vi "MFC-2000 Stage Engine.vi"(0 "MS-2000 Notifier Name":string="MS2000", 11 "COM Port":string[](array[string])) -> ()   [LabVIEW 2020]
uses:
  Stages Controls/Stage Notifier Element.ctl
  Stages Controls/Stage Actions.ctl
  Stages Controls/Stage Status.ctl
  <vilib>/Instr/_visa.llb/VISA Configure Serial Port (Instr).vi
panel:
  in  "XY Velocity (µm/s)":dbl format="%#_4g"
  out "Reply":string
  in  "Command":string
  out "Last Error":errorcluster
  in  "Get Position":bool
  in  "XY Step Size (µm)":dbl format="%#_4g"
  in  "Y Position (µm)":dbl format="%#_4g"
  in  "X Position (µm)":dbl format="%#_4g"
  in  "Home":bool
  in  "Right":bool
  in  "Left":bool
  in  "Down":bool
  in  "Halt":bool
  in  "Up":bool
  in  "Quit":bool
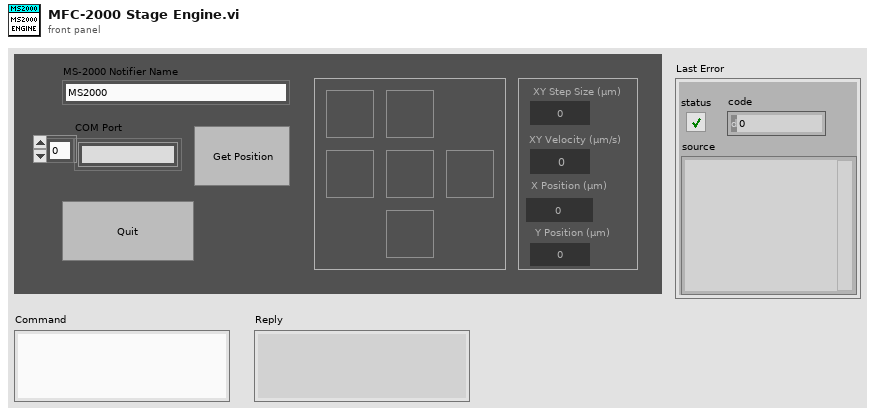
[diagram p1: front panel]
types:
  T1 = typedef "Stage Notifier Element.ctl" = cluster{"Action":T2, "Axis":bool[], "Setpoint":dbl[], "Velocity":dbl, "Cmd Recvd?":bool, "Position":dbl[], "Status":T3, "Misc":variant}
  T2 = typedef "Stage Actions.ctl" = enum16{"Get Position", "MVR", "MOVE", "HALT", "ONTARGET", "ERROR", "REFERENCE", "INIT", "VELOCITY", "STATUS", "EXIT", "HOME", "ZEROPOS", "NANOPOS", "ANALOG", "QUIT"}
  T3 = typedef "Stage Status.ctl" = enum16{"Error", "Abort", "Busy", "On Target"}
  T4 = enum32{"Invalid", "Standard", "Closed", "Hidden", "Minimized", "Maximized"}
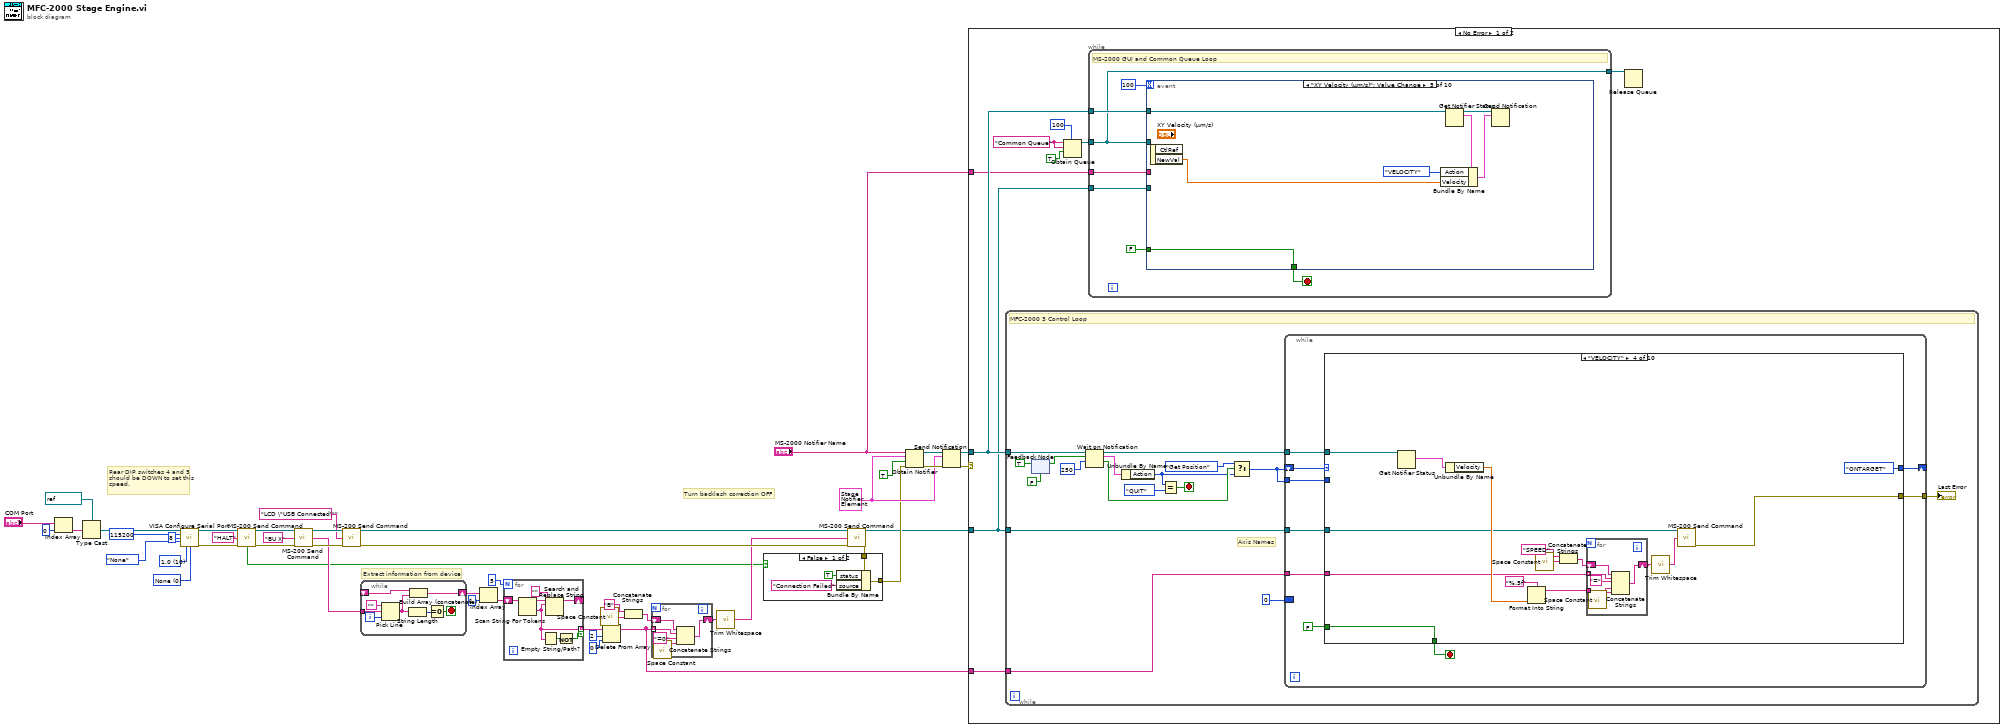
[diagram p0: block diagram]
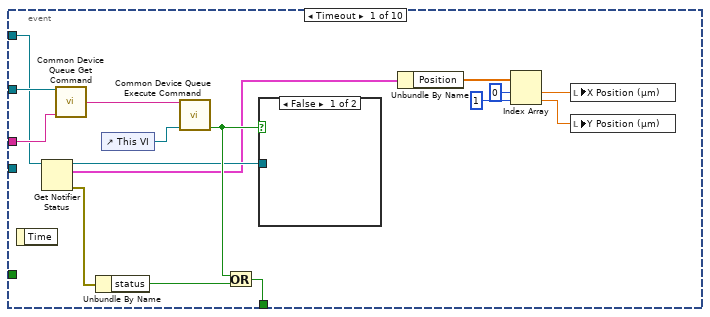
[diagram p3: hidden frame]
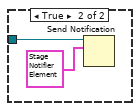
[diagram p4: hidden frame]
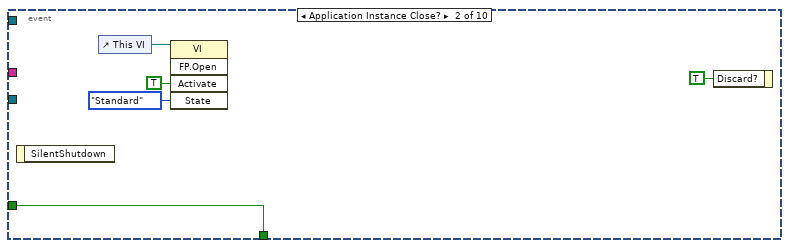
[diagram p5: hidden frame]
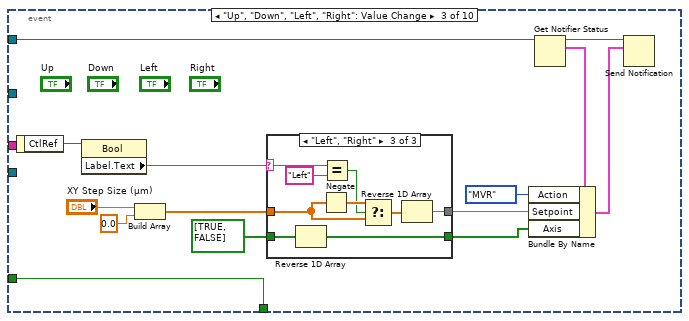
[diagram p6: hidden frame]
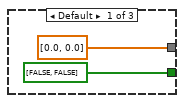
[diagram p7: hidden frame]
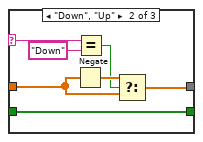
[diagram p8: hidden frame]
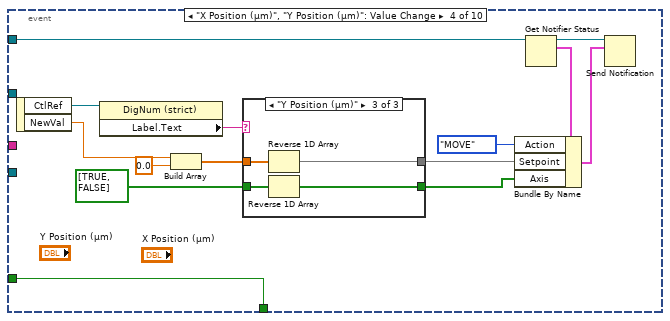
[diagram p9: hidden frame]
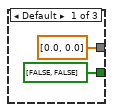
[diagram p10: hidden frame]
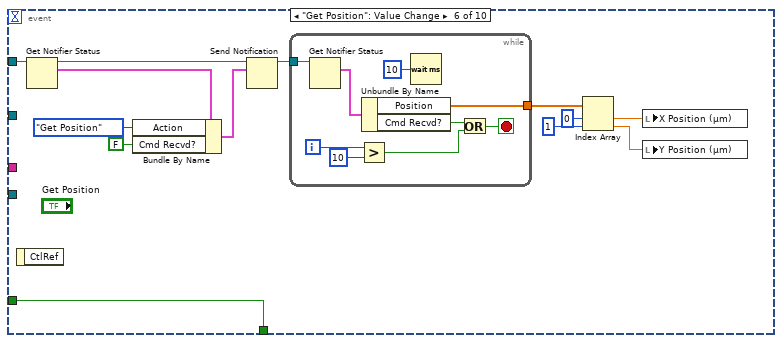
[diagram p12: hidden frame]
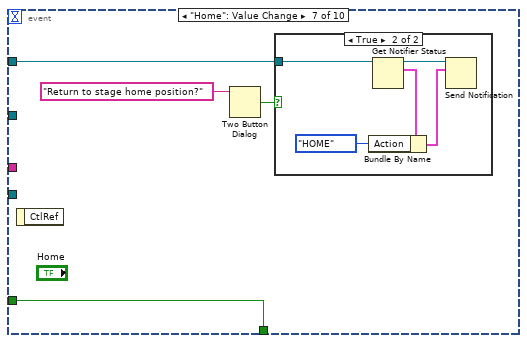
[diagram p13: hidden frame]
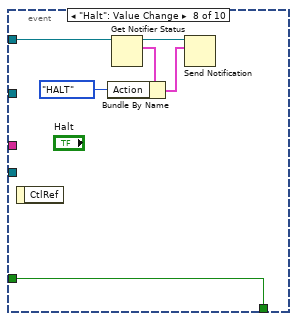
[diagram p15: hidden frame]
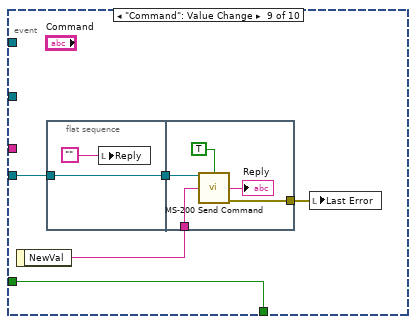
[diagram p16: hidden frame]
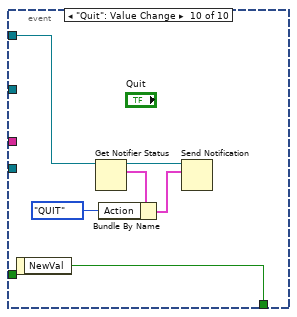
[diagram p17: hidden frame]
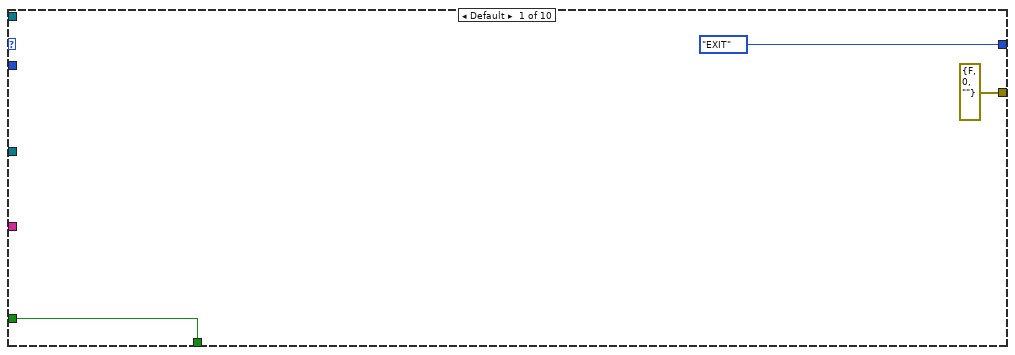
[diagram p18: hidden frame]
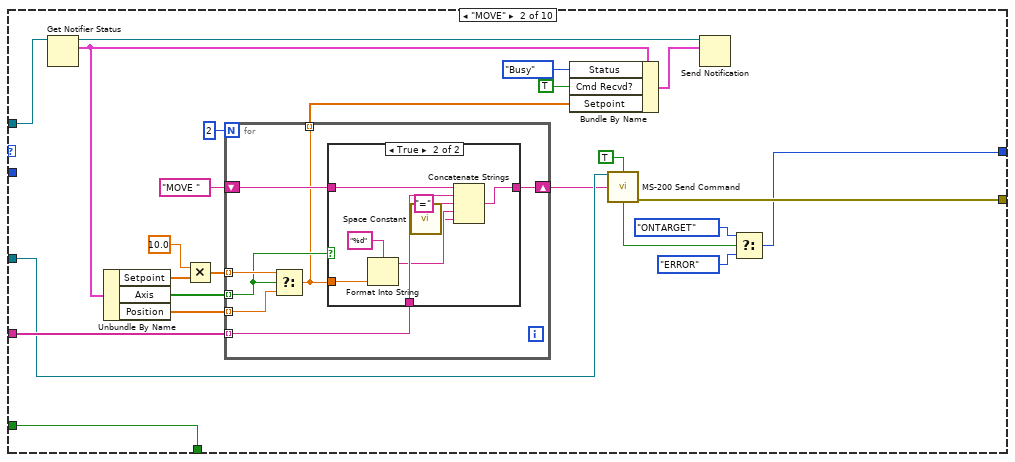
[diagram p19: hidden frame]
diagram:
  w37 = u16 0 items=["None", "XON/XOFF", "RTS/CTS", "XON/XOFF & RTS/CTS", "DTR/DSR", "XON/XOFF & DTR/DSR"] ("flow control (0:none)")
  w39 = u16 10 items=["1.0"=10, "1.5"=15, "2.0"=20] ("stop bits (10: 1 bit)")
  w41 = T1 {"Action"=enum."Get Position", "Axis"=[], "Setpoint"=[], "Velocity"=0.5, "Cmd Recvd?"=FALSE, "Position"=[], "Status"=enum."On Target", "Misc"=variant} ("Stage Status")
  # "Extract information from device"
  # "Turn backlash correction OFF"
  # "Rear DIP switches 4 and 5 should be DOWN to set this speed."
  n1 = Index Array(array="COM Port", index=0) -> (element=w26:string)
  n2 = Type Cast(type=refnum<visa-resource-name> "COM5" ("VISA resource name"), x=w26) -> (*(type *) &x=w25:refnum<visa-resource-name>)
  n3 = call-poly "VISA Configure Serial Port"("VISA resource name"=w25, "baud rate (9600)"=u32 115200, "data bits (8)"=u16 8, "parity (0:none)"=enum16{"None", "Odd", "Even", "Mark", "Space"}."None", "stop bits (10: 1 bit)"=w39, "flow control (0:none)"=w37) -> ("VISA resource name out"=w4:refnum<visa-resource-name>, "error out"=w5:errorcluster)  [unwired: 8 in]
  n4 = call "MS-200 Send Command.vi"("VISA Ref"=w4, "Command"="HALT", "Error In"=w5) -> ("VISA Ref Dup"=w3:refnum<visa-resource-name>, "Cmd Success"=w1:bool, "Error Out"=w2:errorcluster)  [unwired: 9 in, 1 out]
  n5 = call "MS-200 Send Command.vi"("VISA Ref"=w3, "Command"="BU X", "Error In"=w2) -> ("VISA Ref Dup"=w32:refnum<visa-resource-name>, "Reply"=w10:string, "Error Out"=w31:errorcluster)  [unwired: 9 in, 1 out]
  n6 = call "MS-200 Send Command.vi"("VISA Ref"=w32, "Command"="LCD \"USB Connected\"", "Error In"=w31) -> ("VISA Ref Dup"=w23:refnum<visa-resource-name>, "Error Out"=w24:errorcluster)  [unwired: 9 in, 2 out]
  n7 = while {
    tunnel: w10 -> [w54]
    shift-right: [w52] -> w20
    shift-left: _ -> [w51]
    i -> [w47]
    stop <- w48 stop-if-true
    n8 = Pick Line(string ("")="", multi-line string=w54, line index=w47) -> (output string=w49:string)
    n9 = String Length(string=w49) -> (length=w50:i32)
    n10 = Build Array (concatenate)(w51, w49) -> (w52:string[])
    n11 = Equal To 0?(x=w50) -> (x = 0?=w48:bool)
  }
  n12 = Index Array(array=w20, index=1) -> (element=w17:string)
  n13 = for {
    N: 5 -> [_]
    tunnel: [w57] -> w16 mode=indexing if=w55
    shift-right: [w58] -> _
    shift-left: w17 -> [w61]
    n14 = Scan String For Tokens(9:w61) -> (1:w57:string, 3:w60:string)  [unwired: 5 in, 2 out]
    n15 = Empty String/Path?(string/path=w57) -> (empty?=w56:bool)
    n16 = Search and Replace String(input string=w60, search string=w57, replace string="" ("replace string (\"\")")) -> (result string=w58:string)  [unwired: 5 in, 3 out]
    n17 = Not(x=w56) -> (.not. x?=w55:bool)
  }
  n18 = call <vilib>:"Space Constant.vi"() -> ("String"=w12:string)
  n19 = Delete From Array(array=w16, length=2, index=0) -> (array with subset deleted=w7:string[])  [unwired: 1 out]
  n20 = Concatenate Strings("B", w12) -> (w11:string)
  n21 = for {
    tunnel: w7 -> [w66] mode=indexing
    shift-right: [w64] -> w9
    shift-left: w11 -> [w63]
    n22 = call <vilib>:"Space Constant.vi"() -> ("String"=w62:string)
    n23 = Concatenate Strings(w63, w66, "=0" ("string"), w62) -> (w64:string)
  }
  n24 = call <vilib>:"Trim Whitespace.vi"("string"=w9) -> ("trimmed string"=w8:string)  [unwired: 1 in]
  n25 = call "MS-200 Send Command.vi"("VISA Ref"=w23, "Command"=w8, "Error In"=w24) -> ("VISA Ref Dup"=w21:refnum<visa-resource-name>, "Error Out"=w22:errorcluster)  [unwired: 9 in, 2 out]
  n26 = case shown="False" w1 {
    tunnel: w22 -> [w70 w71]
    tunnel: [w67 w71] -> w33
    frame False {
      n27 = Bundle By Name(cluster=w70, "status"=TRUE, "source"="Connection Failed") -> (w67:errorcluster)
    }
    frame True {
    }
  }
  n28 = Obtain Notifier(name (unnamed)="MS-2000 Notifier Name", notification data type=w41, create if not found? (T)=TRUE, error in (no error)=w33) -> (notifier out=w45:refnum<notifier>, error out=w44:errorcluster)  [unwired: 1 out]
  n29 = Send Notification(notification=w41, notifier=w45, error in (no error)=w44) -> (notifier out=w42:refnum<notifier>, error out=w43:errorcluster)
  n30 = case shown="No Error" w43 {
    selector: w43 -> [_ w455]
    tunnel: w42 -> [w77 w456]
    tunnel: w21 -> [w73 w457]
    tunnel: "MS-2000 Notifier Name" -> [w76 _]
    tunnel: w7 -> [w72 _]
    frame No Error {
      w80 = "Common Queue" ("Unique Notifier Name")
      n31 = while {
        tunnel: w77 -> [w243]
        tunnel: w73 -> [w240]
        tunnel: w72 -> [w227]
        stop <- w239 stop-if-true
        # "Axis Names"
        # "MFC-2000 3 Control Loop"
        n32 = feedback-in #1(TRUE ("ignore previous (F)")) -> ()
        n33 = feedback #1(FALSE ("ignore previous (F)")) -> (w234:bool)
        n34 = Wait on Notification(notifier=w243, ignore previous (F)=w234, timeout in ms (-1)=250) -> (notifier out=w242:refnum<notifier>, notification=w238:T1, timed out?=w232:bool)  [unwired: 1 in, 1 out]
        n35 = Unbundle By Name(w238) -> ("Action"=w230:T2)
        n36 = Equal?(x=w230, y=Stage_Actions."QUIT") -> (x = y?=w239:bool)
        n37 = Select(t=Stage_Actions."Get Position", s=w232, f=w230) -> (s? t:f=w229:T2)
        n38 = while {
          tunnel: w242 -> [w252]
          tunnel: w240 -> [w250]
          shift-right: [w249] -> _
          shift-left: w229 -> [w251]
          tunnel: w229 -> [w246]
          border: 0 -> [_]
          tunnel: w227 -> [w245]
          tunnel: [w244] -> w228
          stop <- w247 stop-if-true
          n39 = case shown="\"VELOCITY\"" w251 {
            selector: w251 -> [_ _ _ _ _ _ _ _ w435 _]
            tunnel: w252 -> [_ w275 w311 w335 w358 w373 w401 w428 w437 w448]
            tunnel: w250 -> [_ w264 w299 w334 _ w372 w396 w420 _ w446]
            tunnel: [Stage_Actions."EXIT" ("y") w256 Stage_Actions."ONTARGET" ("y") Stage_Actions."ONTARGET" ("y") Stage_Actions."MOVE" ("y") w375 w398 w425 Stage_Actions."EXIT" ("y") Stage_Actions."QUIT" ("y")] -> w249
            tunnel: FALSE -> [w255 w279 w315 w346 w356 _ w402 w422 _ _]
            tunnel: [w255 w279 w315 w346 w356 w367 w402 w422 TRUE TRUE] -> w247
            tunnel: w246 -> [_ _ _ _ _ _ w397 _ _ _]
            tunnel: w245 -> [_ w266 w301 w333 _ _ w387 _ _ _]
            tunnel: [errorcluster {"status"=FALSE, "code"=0, "source"=""} ("error out") w262 w297 w332 w353 w366 w392 w417 errorcluster {"status"=FALSE, "code"=0, "source"=""} ("Error Out") w443] -> w244
            frame Default {
            }
            frame "MOVE" {
              n40 = Get Notifier Status(notifier=w275) -> (notifier out=w277:refnum<notifier>, current notification=w272:T1)  [unwired: 1 in, 3 out]
              n41 = Unbundle By Name(w272) -> ("Setpoint"=w270:dbl[], "Axis"=w273:bool[], "Position"=w265:dbl[])
              n42 = Multiply(x=10.0, y=w270) -> (x*y=w268:dbl[])
              n43 = for {
                N: 2 -> [_]
                tunnel: w273 -> [w284] mode=indexing
                tunnel: w265 -> [w285] mode=indexing
                tunnel: w268 -> [w286] mode=indexing
                shift-right: [w282] -> w263
                shift-left: "MOVE " -> [w283]
                tunnel: [w280] -> w271 mode=indexing
                tunnel: w266 -> [w281] mode=indexing
                n44 = Select(t=w286, s=w284, f=w285) -> (s? t:f=w280:dbl)
                n45 = case shown="True" w284 {
                  tunnel: w283 -> [w287 w293]
                  tunnel: [w287 w288] -> w282
                  tunnel: w281 -> [_ w292]
                  tunnel: w280 -> [_ w295]
                  frame False {
                  }
                  frame True {
                    n46 = Format Into String(format string="%d", w295) -> (resulting string=w290:string)  [unwired: 2 in, 1 out]
                    n47 = call <vilib>:"Space Constant.vi"() -> ("String"=w289:string)
                    n48 = Concatenate Strings(w293, w292, "=" ("string"), w290, w289) -> (w288:string)
                  }
                }
              }
              n49 = Bundle By Name(cluster=w272, "Status"=Stage_Status."Busy", "Cmd Recvd?"=TRUE, "Setpoint"=w271) -> (w276:T1)
              n50 = call "MS-200 Send Command.vi"("VISA Ref"=w264, "Wait for Reply (T)"=TRUE, "Command"=w263) -> ("Cmd Success"=w259:bool, "Error Out"=w262:errorcluster)  [unwired: 9 in, 2 out]
              n51 = Send Notification(notification=w276, notifier=w277) -> ()  [unwired: 1 in, 2 out]
              n52 = Select(t=Stage_Actions."ONTARGET" ("y"), s=w259, f=Stage_Actions."ERROR") -> (s? t:f=w256:T2)
            }
            frame "MVR" {
              n53 = Get Notifier Status(notifier=w311) -> (notifier out=w313:refnum<notifier>, current notification=w307:T1)  [unwired: 1 in, 3 out]
              n54 = Unbundle By Name(w307) -> ("Setpoint"=w305:dbl[], "Axis"=w308:bool[], "Position"=w300:dbl[])
              n55 = Multiply(x=10.0, y=w305) -> (x*y=w303:dbl[])
              n56 = for {
                N: 2 -> [_]
                tunnel: w308 -> [w320] mode=indexing
                tunnel: w300 -> [w321] mode=indexing
                tunnel: w303 -> [w322] mode=indexing
                shift-right: [w318] -> w298
                shift-left: "MOVREL " -> [w319]
                tunnel: [w316] -> w306 mode=indexing
                tunnel: w301 -> [w317] mode=indexing
                n57 = Select(t=w322, s=w320, f=w321) -> (s? t:f=w316:dbl)
                n58 = case shown="True" w320 {
                  tunnel: w319 -> [w323 w329]
                  tunnel: [w323 w324] -> w318
                  tunnel: w317 -> [_ w328]
                  tunnel: w316 -> [_ w331]
                  frame False {
                  }
                  frame True {
                    n59 = Format Into String(format string="%d", w331) -> (resulting string=w326:string)  [unwired: 2 in, 1 out]
                    n60 = call <vilib>:"Space Constant.vi"() -> ("String"=w325:string)
                    n61 = Concatenate Strings(w329, w328, "=" ("string"), w326, w325) -> (w324:string)
                  }
                }
              }
              n62 = Bundle By Name(cluster=w307, "Status"=Stage_Status."Busy", "Cmd Recvd?"=TRUE, "Setpoint"=w306) -> (w312:T1)
              n63 = call "MS-200 Send Command.vi"("VISA Ref"=w299, "Command"=w298) -> ("Error Out"=w297:errorcluster)  [unwired: 10 in, 3 out]
              n64 = Send Notification(notification=w312, notifier=w313) -> ()  [unwired: 1 in, 2 out]
            }
            frame "VELOCITY" {
              n65 = Get Notifier Status(notifier=w335) -> (current notification=w339:T1)  [unwired: 1 in, 4 out]
              n66 = Unbundle By Name(w339) -> ("Velocity"=w336:dbl)
              n67 = Format Into String(format string="%.5f", w336) -> (resulting string=w337:string)  [unwired: 2 in, 1 out]
              n68 = call <vilib>:"Space Constant.vi"() -> ("String"=w343:string)
              n69 = Concatenate Strings("SPEED", w343) -> (w342:string)
              n70 = for {
                tunnel: w333 -> [w352] mode=indexing
                shift-right: [w351] -> w341
                shift-left: w342 -> [w350]
                tunnel: w337 -> [w347]
                n71 = call <vilib>:"Space Constant.vi"() -> ("String"=w349:string)
                n72 = Concatenate Strings(w350, w352, "=" ("string"), w347, w349) -> (w351:string)
              }
              n73 = call <vilib>:"Trim Whitespace.vi"("string"=w341) -> ("trimmed string"=w340:string)  [unwired: 1 in]
              n74 = call "MS-200 Send Command.vi"("VISA Ref"=w334, "Command"=w340) -> ("Error Out"=w332:errorcluster)  [unwired: 10 in, 3 out]
            }
            frame "HOME" {
              n75 = Get Notifier Status(notifier=w358) -> (notifier out=w360:refnum<notifier>, current notification=w361:T1)  [unwired: 1 in, 3 out]
              n76 = Bundle By Name(cluster=w361, "Setpoint"=dbl[] [0.0, 0.0], "Axis"=bool[] [TRUE, TRUE], "Status"=Stage_Status."Busy") -> (w359:T1)
              n77 = Send Notification(notification=w359, notifier=w360) -> (error out=w353:errorcluster)  [unwired: 1 in, 1 out]
            }
            frame "ONTARGET" {
              n78 = feedback #2() -> (w378:i32)
              n79 = call "MS-200 Send Command.vi"("VISA Ref"=w372, "Command"="/") -> ("Reply"=w370:string, "Error Out"=w366:errorcluster)  [unwired: 10 in, 2 out]
              n80 = Increment(x=w378) -> (x+1=w377:i32)
              n81 = feedback-in #2(w377) -> ()
              n82 = Equal?(x="N", y=w370) -> (x = y?=w368:bool)
              n83 = Greater?(x=w377, y=250) -> (0:w367:bool)
              n84 = Wait (ms)(milliseconds to wait=u32 50) -> ()  [unwired: 1 out]
              n85 = Select(t=Stage_Actions."EXIT" ("y"), s=w368, f=Stage_Actions."Get Position" ("y")) -> (s? t:f=w364:T2)
              n86 = Select(t=Stage_Status."On Target" ("Status"), s=w368, f=Stage_Status."Busy" ("Status")) -> (s? t:f=w379:T3)
              n87 = Get Notifier Status(notifier=w373) -> (notifier out=w383:refnum<notifier>, current notification=w384:T1)  [unwired: 1 in, 3 out]
              n88 = Bundle By Name(cluster=w384, "Status"=w379) -> (w382:T1)
              n89 = Send Notification(notification=w382, notifier=w383) -> ()  [unwired: 1 in, 2 out]
              n90 = Select(t=Stage_Actions."ERROR" ("f"), s=w367, f=w364) -> (s? t:f=w375:T2)
            }
            frame "Get Position" {
              n91 = call <vilib>:"Space Constant.vi"() -> ("String"=w390:string)
              n92 = Concatenate Strings("WHERE", w390) -> (w389:string)
              n93 = for {
                tunnel: w387 -> [w407] mode=indexing
                shift-right: [w406] -> w388
                shift-left: w389 -> [w405]
                n94 = call <vilib>:"Space Constant.vi"() -> ("String"=w404:string)
                n95 = Concatenate Strings(w405, w407, w404) -> (w406:string)
              }
              n96 = call <vilib>:"Trim Whitespace.vi"("string"=w388) -> ("trimmed string"=w386:string)  [unwired: 1 in]
              n97 = call "MS-200 Send Command.vi"("VISA Ref"=w396, "Command"=w386) -> ("Reply"=w394:string, "Error Out"=w395:errorcluster)  [unwired: 10 in, 2 out]
              n98 = call "MS-2000 Read Positions.vi"("WHERE Reply"=w394, "Error In"=w395) -> ("Positions um"=w393:dbl[], "Error Out"=w392:errorcluster)  [unwired: 11 in, 1 out]
              n99 = Get Notifier Status(notifier=w401) -> (notifier out=w403:refnum<notifier>, current notification=w400:T1)  [unwired: 1 in, 3 out]
              n100 = case shown="Default" w397 {
                tunnel: w400 -> [w411 w416]
                tunnel: [w410 w415] -> w399
                tunnel: w393 -> [w409 w414]
                tunnel: [Stage_Actions."ONTARGET" ("y") Stage_Actions."EXIT" ("y")] -> w398
                frame Default {
                  n101 = Bundle By Name(cluster=w411, "Position"=w409) -> (w410:T1)
                }
                frame "Get Position", "HALT" {
                  n102 = Bundle By Name(cluster=w416, "Position"=w414, "Cmd Recvd?"=TRUE) -> (w415:T1)
                }
              }
              n103 = Send Notification(notification=w399, notifier=w403) -> ()  [unwired: 1 in, 2 out]
            }
            frame "HALT" {
              n104 = call "MS-200 Send Command.vi"("VISA Ref"=w420, "Command"="HALT") -> ("Cmd Success"=w418:bool, "Error Out"=w417:errorcluster)  [unwired: 10 in, 2 out]
              n105 = Select(t=Stage_Status."Abort" ("Status"), s=w418, f=Stage_Status."Error" ("Status")) -> (s? t:f=w421:T3)
              n106 = Select(t=Stage_Actions."Get Position" ("y"), s=w418, f=Stage_Actions."ERROR" ("y")) -> (s? t:f=w425:T2)
              n107 = Get Notifier Status(notifier=w428) -> (notifier out=w431:refnum<notifier>, current notification=w432:T1)  [unwired: 1 in, 3 out]
              n108 = Bundle By Name(cluster=w432, "Status"=w421, "Cmd Recvd?"=TRUE) -> (w430:T1)
              n109 = Send Notification(notification=w430, notifier=w431) -> ()  [unwired: 1 in, 2 out]
            }
            frame "ERROR", "EXIT" {
              n110 = case shown="\"ERROR\"" w435 {
                tunnel: w437 -> [_ w442]
                frame Default {
                }
                frame "ERROR" {
                  n111 = Get Notifier Status(notifier=w442) -> (notifier out=w439:refnum<notifier>, current notification=w441:T1)  [unwired: 1 in, 3 out]
                  n112 = Bundle By Name(cluster=w441, "Status"=Stage_Status."Error") -> (w438:T1)
                  n113 = Send Notification(notification=w438, notifier=w439) -> ()  [unwired: 1 in, 2 out]
                }
              }
            }
            frame "QUIT" {
              n114 = Release Notifier(notifier=w448, force destroy? (F)=TRUE) -> ()  [unwired: 1 in, 3 out]
              n115 = VISA Close(VISA resource name=w446) -> (error out=w443:errorcluster)  [unwired: 1 in]
            }
          }
        }
        "Last Error" <- w228
      }
      n116 = Obtain Queue(max queue size (-1, unlimited)=100, name (unnamed)=w80, element data type=w80, create if not found? (T)=TRUE) -> (queue out=w78:refnum<queue>)  [unwired: 1 in, 2 out]
      n117 = while {
        tunnel: w78 -> [w82]
        tunnel: w76 -> [w85]
        tunnel: w77 -> [w86]
        tunnel: [w82] -> w74
        tunnel: w73 -> [w81]
        stop <- w84 stop-if-true
        # "MS-2000 GUI and Common Queue Loop"
        n118 = event shown="[4] \"XY Velocity (µm/s)\": Value Change" {
          selector: _ -> [_ _ _ _ _ _ _ _ _ _]
          dyn-events: _ -> [_ _ _ _ _ _ _ _ _ _]
          timeout: 100 -> [_ _ _ _ _ _ _ _ _ _]
          tunnel: w82 -> [w97 _ _ _ _ _ _ _ _ _]
          tunnel: w86 -> [w94 _ w117 w149 w170 w183 w194 w207 _ w226]
          tunnel: w85 -> [w96 _ _ _ _ _ _ _ _ _]
          tunnel: [w95 w110 w120 w156 w171 w184 w196 w208 w213 w222] -> w84
          tunnel: FALSE -> [_ w110 w120 w156 w171 w184 w196 w208 w213 _]
          tunnel: w81 -> [_ _ _ _ _ _ _ _ w210 _]
          event Timeout {
            n119 = event-data() -> ()  [unwired: 1 in, 1 out]
            n120 = Get Notifier Status(notifier=w94) -> (notifier out=w98:refnum<notifier>, current notification=w88:T1, error out=w103:errorcluster)  [unwired: 1 in, 2 out]
            n121 = call "Common Device Queue Get Command.vi"("Common Queue"=w97, "Notifier Name"=w96) -> ("Command"=w102:string)  [unwired: 12 in, 1 out]
            n122 = Unbundle By Name(w103) -> ("status"=w100:bool)
            n123 = control-ref of="This VI"() -> (w101:refnum<vi>)
            n124 = call "Common Device Queue Execute Command.vi"("Common Command"=w102, "VI Refnum"=w101) -> ("Quit?"=w99:bool)  [unwired: 12 in, 1 out]
            n125 = Or(x=w99, y=w100) -> (x .or. y?=w95:bool)
            n126 = case shown="False" w99 {
              tunnel: w98 -> [_ w105]
              frame False {
              }
              frame True {
                n127 = Send Notification(notification=T1 {"Action"=enum."QUIT", "Axis"=[], "Setpoint"=[], "Velocity"=0.5, "Cmd Recvd?"=FALSE, "Position"=[], "Status"=enum."Error", "Misc"=variant} ("Stage Status"), notifier=w105) -> ()  [unwired: 1 in, 2 out]
              }
            }
            n128 = Unbundle By Name(w88) -> ("Position"=w89:dbl[])
            n129 = Index Array(array=w89, index #1=0 ("index"), index #2=1 ("index")) -> (element #1=w93:dbl, element #2=w92:dbl)
            n130 = local write "X Position (µm)"(w93) -> ()
            n131 = local write "Y Position (µm)"(w92) -> ()
          }
          event Application Instance Close? {
            n132 = event-data() -> ()  [unwired: 1 in, 1 out]
            n133 = control-ref of="This VI"() -> (w107:refnum<vi>)
            n134 = invoke class="VI" method="FP.Open"(reference=w107, "Activate"=TRUE ("Activate?"), "State"=T4."Standard") -> ()  [unwired: 2 in, 5 out]
            n135 = event-data("Discard?"=TRUE) -> ()  [unwired: 1 in, 1 out]
          }
          event "Up", "Down", "Left", "Right": Value Change {
            n136 = event-data() -> ("CtlRef"=w119:refnum<vi>)  [unwired: 1 in]
            n137 = property class="Bool"(reference=w119) -> ("Label.Text"=w124:string)  [unwired: 1 in, 2 out]
            n138 = Build Array("XY Step Size (µm)", 0.0 ("element")) -> (w122:dbl[])
            n139 = case shown="\"Left\", \"Right\"" w124 {
              selector: w124 -> [_ w133 w139]
              tunnel: w122 -> [_ w130 w138]
              tunnel: bool[] [TRUE, FALSE] -> [_ w127 w136]
              tunnel: [dbl[] [0.0, 0.0] w129 w135] -> w115
              tunnel: [bool[] [FALSE, FALSE] w127 w134] -> w114
              frame Default {
              }
              frame "Down", "Up" {
                n140 = Negate(x=w130) -> (-x=w131:dbl[])
                n141 = Equal?(x=w133, y="Down") -> (x = y?=w128:bool)
                n142 = Select(t=w131, s=w128, f=w130) -> (s? t:f=w129:dbl[])
              }
              frame "Left", "Right" {
                n143 = Reverse 1D Array(array=w136) -> (reversed array=w134:bool[])
                n144 = Negate(x=w138) -> (-x=w141:dbl[])
                n145 = Equal?(x=w139, y="Left") -> (x = y?=w140:bool)
                n146 = Select(t=w141, s=w140, f=w138) -> (s? t:f=w137:dbl[])
                n147 = Reverse 1D Array(array=w137) -> (reversed array=w135:dbl[])
              }
            }
            n148 = Get Notifier Status(notifier=w117) -> (notifier out=w112:refnum<notifier>, current notification=w116:T1)  [unwired: 1 in, 3 out]
            n149 = Bundle By Name(cluster=w116, "Action"=Stage_Actions."MVR", "Setpoint"=w115, "Axis"=w114) -> (w111:T1)
            n150 = Send Notification(notification=w111, notifier=w112) -> ()  [unwired: 1 in, 2 out]
          }
          event "X Position (µm)", "Y Position (µm)": Value Change {
            n151 = event-data() -> ("CtlRef"=w151:refnum<vi>, "NewVal"=w150:dbl)  [unwired: 1 in]
            n152 = property class="DigNum (strict)"(reference=w151) -> ("Label.Text"=w154:string)  [unwired: 1 in, 2 out]
            n153 = Build Array(w150, 0.0 ("element")) -> (w155:dbl[])
            n154 = case shown="\"Y Position (µm)\"" w154 {
              tunnel: w155 -> [_ w160 w164]
              tunnel: bool[] [TRUE, FALSE] -> [_ w159 w163]
              tunnel: [dbl[] [0.0, 0.0] w160 w162] -> w146
              tunnel: [bool[] [FALSE, FALSE] w159 w161] -> w145
              frame Default {
              }
              frame "X Position (µm)" {
              }
              frame "Y Position (µm)" {
                n155 = Reverse 1D Array(array=w164) -> (reversed array=w162:dbl[])
                n156 = Reverse 1D Array(array=w163) -> (reversed array=w161:bool[])
              }
            }
            n157 = Get Notifier Status(notifier=w149) -> (notifier out=w148:refnum<notifier>, current notification=w147:T1)  [unwired: 1 in, 3 out]
            n158 = Bundle By Name(cluster=w147, "Action"=Stage_Actions."MOVE", "Setpoint"=w146, "Axis"=w145) -> (w143:T1)
            n159 = Send Notification(notification=w143, notifier=w148) -> ()  [unwired: 1 in, 2 out]
          }
          event "XY Velocity (µm/s)": Value Change {
            n160 = event-data() -> ("NewVal"=w165:dbl)  [unwired: 1 in, 1 out]
            n161 = Get Notifier Status(notifier=w170) -> (notifier out=w169:refnum<notifier>, current notification=w168:T1)  [unwired: 1 in, 3 out]
            n162 = Bundle By Name(cluster=w168, "Action"=Stage_Actions."VELOCITY", "Velocity"=w165) -> (w166:T1)
            n163 = Send Notification(notification=w166, notifier=w169) -> ()  [unwired: 1 in, 2 out]
          }
          event "Get Position": Value Change {
            n164 = event-data() -> ()  [unwired: 1 in, 1 out]
            n165 = Get Notifier Status(notifier=w183) -> (notifier out=w182:refnum<notifier>, current notification=w181:T1)  [unwired: 1 in, 3 out]
            n166 = Bundle By Name(cluster=w181, "Action"=Stage_Actions."Get Position", "Cmd Recvd?"=FALSE) -> (w178:T1)
            n167 = Send Notification(notification=w178, notifier=w182) -> (notifier out=w177:refnum<notifier>)  [unwired: 1 in, 1 out]
            n168 = while {
              tunnel: w177 -> [w193]
              tunnel: [w185] -> w176
              i -> [w189]
              stop <- w186 stop-if-true
              n169 = Get Notifier Status(notifier=w193) -> (current notification=w192:T1)  [unwired: 1 in, 4 out]
              n170 = Greater?(x=w189, y=10) -> (0:w187:bool)
              n171 = Unbundle By Name(w192) -> ("Position"=w185:dbl[], "Cmd Recvd?"=w188:bool)
              n172 = Wait (ms)(milliseconds to wait=u32 10) -> ()  [unwired: 1 out]
              n173 = Or(x=w188, y=w187) -> (x .or. y?=w186:bool)
            }
            n174 = Index Array(array=w176, index #1=0 ("index"), index #2=1 ("index")) -> (element #1=w173:dbl, element #2=w172:dbl)
            n175 = local write "X Position (µm)"(w173) -> ()
            n176 = local write "Y Position (µm)"(w172) -> ()
          }
          event "Home": Value Change {
            n177 = event-data() -> ()  [unwired: 1 in, 1 out]
            n178 = Two Button Dialog(message="Return to stage home position?") -> (T button?=w195:bool)  [unwired: 2 in]
            n179 = case shown="True" w195 {
              tunnel: w194 -> [_ w202]
              frame False {
              }
              frame True {
                n180 = Get Notifier Status(notifier=w202) -> (notifier out=w201:refnum<notifier>, current notification=w200:T1)  [unwired: 1 in, 3 out]
                n181 = Bundle By Name(cluster=w200, "Action"=Stage_Actions."HOME") -> (w199:T1)
                n182 = Send Notification(notification=w199, notifier=w201) -> ()  [unwired: 1 in, 2 out]
              }
            }
          }
          event "Halt": Value Change {
            n183 = event-data() -> ()  [unwired: 1 in, 1 out]
            n184 = Get Notifier Status(notifier=w207) -> (notifier out=w206:refnum<notifier>, current notification=w205:T1)  [unwired: 1 in, 3 out]
            n185 = Bundle By Name(cluster=w205, "Action"=Stage_Actions."HALT") -> (w204:T1)
            n186 = Send Notification(notification=w204, notifier=w206) -> ()  [unwired: 1 in, 2 out]
          }
          event "Command": Value Change {
            n187 = event-data() -> ("NewVal"=w209:string)  [unwired: 1 in]
            n188 = flat-sequence {
              tunnel: w210 -> [w215]
              tunnel: [w215] -> w212
              tunnel: w212 -> [w220]
              tunnel: [w219] -> w211
              tunnel: w209 -> [w216]
              frame #0 {
                n189 = local write "Reply"("") -> ()
              }
              frame #1 {
                n190 = call "MS-200 Send Command.vi"("VISA Ref"=w220, "Wait for Reply (T)"=TRUE, "Command"=w216) -> ("Reply"=→"Reply":string, "Error Out"=w219:errorcluster)  [unwired: 9 in, 2 out]
              }
            }
            n191 = local write "Last Error"(w211) -> ()
          }
          event "Quit": Value Change {
            n192 = event-data() -> ("NewVal"=w222:bool)  [unwired: 1 in]
            n193 = Get Notifier Status(notifier=w226) -> (notifier out=w225:refnum<notifier>, current notification=w224:T1)  [unwired: 1 in, 3 out]
            n194 = Bundle By Name(cluster=w224, "Action"=Stage_Actions."QUIT") -> (w223:T1)
            n195 = Send Notification(notification=w223, notifier=w225) -> ()  [unwired: 1 in, 2 out]
          }
        }
      }
      n196 = Release Queue(queue=w74) -> ()  [unwired: 2 in, 3 out]
    }
    frame Error {
      n197 = VISA Close(VISA resource name=w457) -> ()  [unwired: 1 in, 1 out]
      n198 = Release Notifier(notifier=w456, force destroy? (F)=TRUE, error in (no error)=w455) -> (error out=w453:errorcluster)  [unwired: 2 out]
      n199 = Unbundle By Name(w453) -> ("source"=w450:string)
      n200 = Concatenate Strings("Pro Scan 3 Error", "\r", w450) -> (w449:string)
      n201 = One Button Dialog(message=w449) -> ()  [unwired: 1 in, 1 out]
    }
  }
